vi "Configure Math Function Characteristics.vi"(0 "VISA resource name":refnum<visa-resource-name>, 1 "Vertical Offset (0.0)":dbl, 2 "Vertical Scale (10.0)":dbl=10.0, 3 "Integrate DC Offset (0.0)":dbl, 5 "Math Operation (0: Add)":i32(ring) items=["Add", "Subtract", "Multiply", "Integrate", "Diff", "FFT", "SQRT", "Magnify", "Absolute", "Square", "LN", "LOG", "EXP", "TEN", "Lowpass", "Highpass", "Divide", "Linear", "Trend", "Btiming", "Bstate", "Envelope", "Smoothing", "Max Hold", "Min Hold", "Average", "Clock Recovery", "Peak", "FFT Phase", "MAX", "MIN", "Bandpass", "Serchart"], 7 "GOFT Math Operation (0: Add)":i32(ring) items=["Add", "Subtract", "Multiply"], 9 "Enable Display (T: Enable)":bool=TRUE, 11 "error in (no error)":errorcluster, 12 "Vertical Range (8.0 V)":dbl=8.0, 13 "Vertical Scale Units (0: V)":i32(ring) items=["V", "dB"], 14 "Math Function Index (1: Math Function 1)":i32(ring)=1 items=["Math Function 1"=1, "Math Function 2"=2, "Math Function 3"=3, "Math Function 4"=4]) -> (4 "VISA resource name out":refnum<visa-resource-name>, 15 "error out":errorcluster)   [LabVIEW 2017, in "Agilent 2000 3000 X-Series.lvlib"]
doc: "Configures the math function."
uses:
  Agilent 2000 3000 X-Series.lvlib
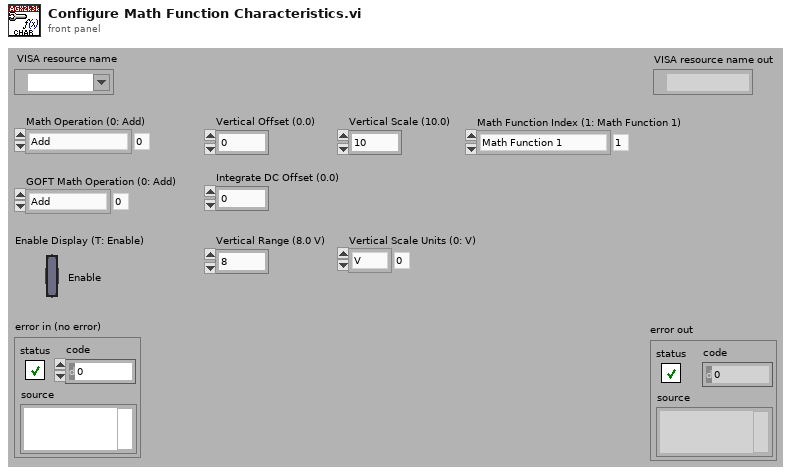
[diagram p1: front panel]
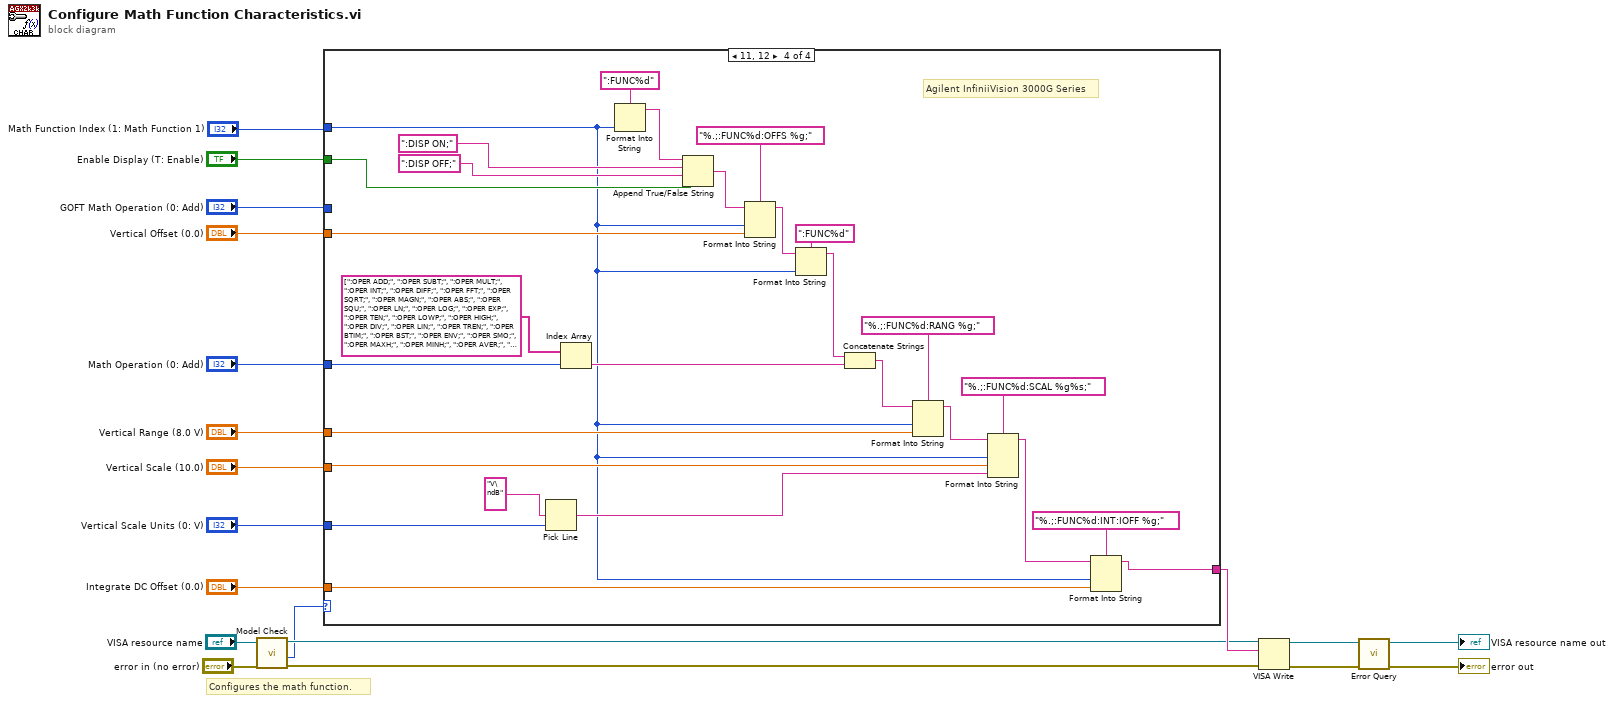
[diagram p0: block diagram]
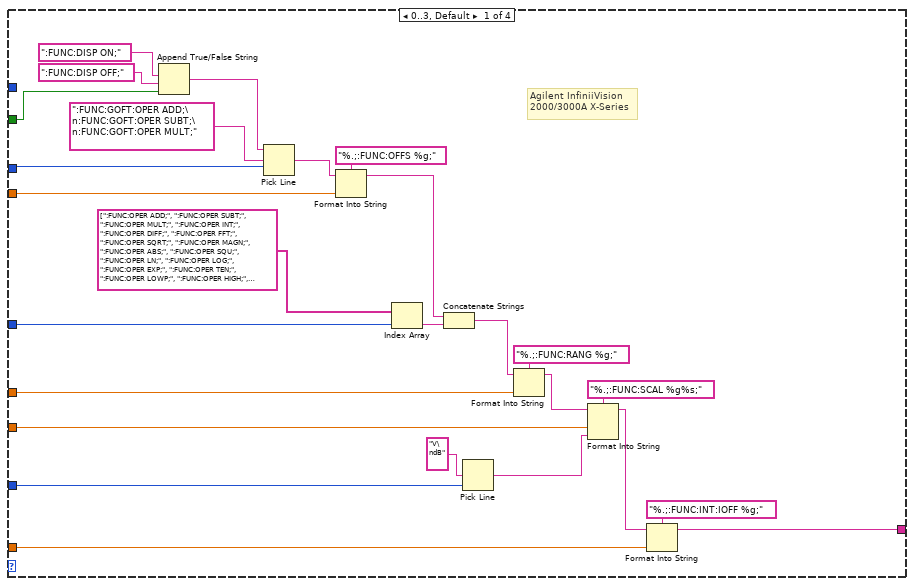
[diagram p2: hidden frame]
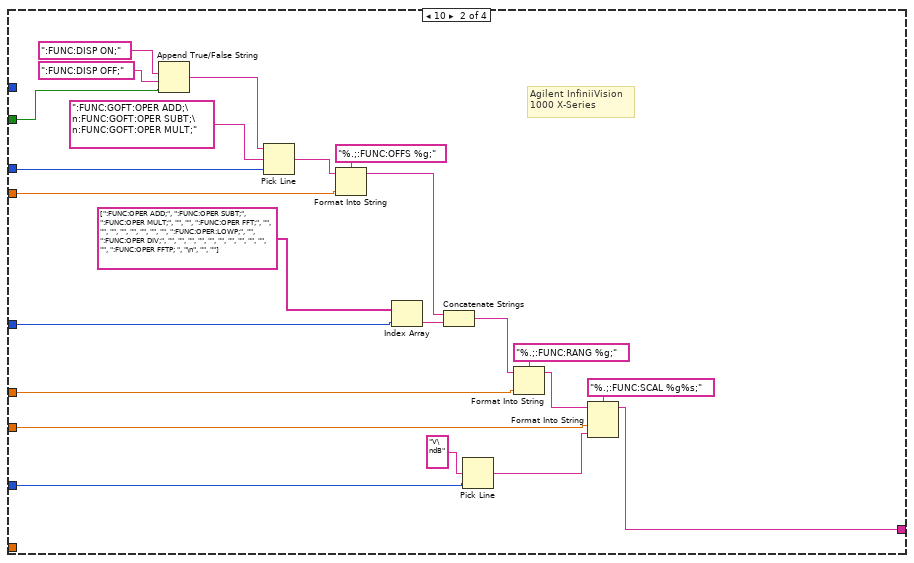
[diagram p3: hidden frame]
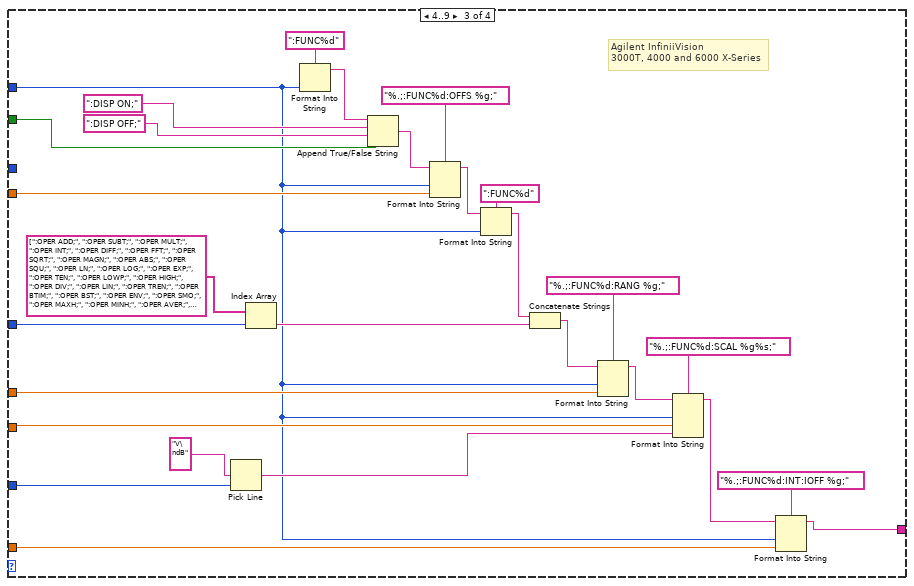
[diagram p4: hidden frame]
diagram:
  # "Configures the math function."
  n1 = call "Model Check.vi"("error in (no error)"="error in (no error)", "VISA resource name"="VISA resource name") -> ("error out"=w2:errorcluster, "Model"=w1:i32, "VISA resource name out"=w3:refnum<visa-resource-name>)  [unwired: 7 out]
  n2 = case shown="11, 12" w1 {
    tunnel: "Enable Display (T: Enable)" -> [w30 w53 w82 w110]
    tunnel: "GOFT Math Operation (0: Add)" -> [w29 w46 _ _]
    tunnel: "Vertical Offset (0.0)" -> [w28 w52 w81 w109]
    tunnel: "Math Operation (0: Add)" -> [w27 w51 w72 w100]
    tunnel: "Vertical Range (8.0 V)" -> [w26 w50 w80 w108]
    tunnel: "Vertical Scale (10.0)" -> [w25 w49 w77 w105]
    tunnel: "Vertical Scale Units (0: V)" -> [w24 w48 w78 w106]
    tunnel: "Integrate DC Offset (0.0)" -> [w23 _ w76 w104]
    tunnel: "Math Function Index (1: Math Function 1)" -> [_ _ w74 w102]
    tunnel: [w22 w47 w71 w99] -> w6
    frame 0..3, Default {
      # "Agilent InfiniiVision\n2000/3000A X-Series"
      n3 = Append True/False String(1:w30, 2:":FUNC:DISP OFF;", 3:":FUNC:DISP ON;") -> (0:w42:string)  [unwired: 1 out]
      n4 = Pick Line(string ("")=w42, multi-line string=":FUNC:GOFT:OPER ADD;\n:FUNC:GOFT:OPER SUBT;\n:FUNC:GOFT:OPER MULT;", line index=w29) -> (output string=w41:string)
      n5 = Format Into String(format string="%.;:FUNC:OFFS %g;", initial string=w41, w28) -> (resulting string=w34:string)  [unwired: 1 in, 1 out]
      n6 = Index Array(array=string[] [":FUNC:OPER ADD;", ":FUNC:OPER SUBT;", ":FUNC:OPER MULT;", ":FUNC:OPER INT;", ":FUNC:OPER DIFF;", ":FUNC:OPER FFT;", ":FUNC:OPER SQRT;", ":FUNC:OPER MAGN;", ":FUNC:OPER ABS;", ":FUNC:OPER SQU;", ":FUNC:OPER LN;", ":FUNC:OPER LOG;", ":FUNC:OPER EXP;", ":FUNC:OPER TEN;", ":FUNC:OPER LOWP;", ":FUNC:OPER HIGH;", ":FUNC:OPER DIV;", ":FUNC:OPER LIN;", ":FUNC:OPER TREN;", ":FUNC:OPER BTIM;", ":FUNC:OPER BST;", "", "", "", "", "", "", "", "\n", "", ""], index=w27) -> (element=w20:string)
      n7 = Concatenate Strings(w34, w20) -> (w33:string)
      n8 = Pick Line(multi-line string="V\ndB", line index=w24) -> (output string=w35:string)  [unwired: 1 out]
      n9 = Format Into String(format string="%.;:FUNC:RANG %g;", initial string=w33, w26) -> (resulting string=w37:string)  [unwired: 1 in, 1 out]
      n10 = Format Into String(format string="%.;:FUNC:SCAL %g%s;", initial string=w37, w25, w35) -> (resulting string=w31:string)  [unwired: 1 in, 1 out]
      n11 = Format Into String(format string="%.;:FUNC:INT:IOFF %g;", initial string=w31, w23) -> (resulting string=w22:string)  [unwired: 1 in, 1 out]
    }
    frame 10 {
      # "Agilent InfiniiVision\n1000 X-Series"
      n12 = Append True/False String(1:w53, 2:":FUNC:DISP OFF;", 3:":FUNC:DISP ON;") -> (0:w65:string)  [unwired: 1 out]
      n13 = Pick Line(string ("")=w65, multi-line string=":FUNC:GOFT:OPER ADD;\n:FUNC:GOFT:OPER SUBT;\n:FUNC:GOFT:OPER MULT;", line index=w46) -> (output string=w64:string)
      n14 = Format Into String(format string="%.;:FUNC:OFFS %g;", initial string=w64, w52) -> (resulting string=w57:string)  [unwired: 1 in, 1 out]
      n15 = Index Array(array=string[] [":FUNC:OPER ADD;", ":FUNC:OPER SUBT;", ":FUNC:OPER MULT;", "", "", ":FUNC:OPER FFT;", "", "", "", "", "", "", "", "", ":FUNC:OPER:LOWP;", "", ":FUNC:OPER DIV;", "", "", "", "", "", "", "", "", "", "", "", ":FUNC:OPER FFTP; ", "\n", "", ""], index=w51) -> (element=w54:string)
      n16 = Concatenate Strings(w57, w54) -> (w56:string)
      n17 = Pick Line(multi-line string="V\ndB", line index=w48) -> (output string=w58:string)  [unwired: 1 out]
      n18 = Format Into String(format string="%.;:FUNC:RANG %g;", initial string=w56, w50) -> (resulting string=w60:string)  [unwired: 1 in, 1 out]
      n19 = Format Into String(format string="%.;:FUNC:SCAL %g%s;", initial string=w60, w49, w58) -> (resulting string=w47:string)  [unwired: 1 in, 1 out]
    }
    frame 4..9 {
      # "Agilent InfiniiVision\n3000T, 4000 and 6000 X-Series"
      n20 = Pick Line(multi-line string="V\ndB", line index=w78) -> (output string=w79:string)  [unwired: 1 out]
      n21 = Index Array(array=string[] [":OPER ADD;", ":OPER SUBT;", ":OPER MULT;", ":OPER INT;", ":OPER DIFF;", ":OPER FFT;", ":OPER SQRT;", ":OPER MAGN;", ":OPER ABS;", ":OPER SQU;", ":OPER LN;", ":OPER LOG;", ":OPER EXP;", ":OPER TEN;", ":OPER LOWP;", ":OPER HIGH;", ":OPER DIV;", ":OPER LIN;", ":OPER TREN;", ":OPER BTIM;", ":OPER BST;", ":OPER ENV;", ":OPER SMO;", ":OPER MAXH;", ":OPER MINH;", ":OPER AVER;", ":OPER CLOCK;", ":OPER PEAK; ", ":OPER FFTP;\n", ":OPER MAX;", ":OPER MIN;"], index=w72) -> (element=w88:string)
      n22 = Format Into String(format string=":FUNC%d", w74) -> (resulting string=w83:string)  [unwired: 2 in, 1 out]
      n23 = Append True/False String(1:w82, 2:":DISP OFF;", 3:":DISP ON;", 4:w83) -> (0:w70:string)
      n24 = Format Into String(format string="%.;:FUNC%d:OFFS %g;", initial string=w70, w74, w81) -> (resulting string=w69:string)  [unwired: 1 in, 1 out]
      n25 = Format Into String(format string=":FUNC%d", initial string=w69, w74) -> (resulting string=w73:string)  [unwired: 1 in, 1 out]
      n26 = Concatenate Strings(w73, w88) -> (w87:string)
      n27 = Format Into String(format string="%.;:FUNC%d:RANG %g;", initial string=w87, w74, w80) -> (resulting string=w91:string)  [unwired: 1 in, 1 out]
      n28 = Format Into String(format string="%.;:FUNC%d:SCAL %g%s;", initial string=w91, w74, w77, w79) -> (resulting string=w85:string)  [unwired: 1 in, 1 out]
      n29 = Format Into String(format string="%.;:FUNC%d:INT:IOFF %g;", initial string=w85, w74, w76) -> (resulting string=w71:string)  [unwired: 1 in, 1 out]
    }
    frame 11, 12 {
      # "Agilent InfiniiVision 3000G Series"
      n30 = Pick Line(multi-line string="V\ndB", line index=w106) -> (output string=w107:string)  [unwired: 1 out]
      n31 = Index Array(array=string[] [":OPER ADD;", ":OPER SUBT;", ":OPER MULT;", ":OPER INT;", ":OPER DIFF;", ":OPER FFT;", ":OPER SQRT;", ":OPER MAGN;", ":OPER ABS;", ":OPER SQU;", ":OPER LN;", ":OPER LOG;", ":OPER EXP;", ":OPER TEN;", ":OPER LOWP;", ":OPER HIGH;", ":OPER DIV;", ":OPER LIN;", ":OPER TREN;", ":OPER BTIM;", ":OPER BST;", ":OPER ENV;", ":OPER SMO;", ":OPER MAXH;", ":OPER MINH;", ":OPER AVER;", "", ":OPER PEAK; ", ":OPER FFTP;\n", ":OPER MAX;", ":OPER MIN;", ":OPER BAND; ", ":OPER SERC; "], index=w100) -> (element=w116:string)
      n32 = Format Into String(format string=":FUNC%d", w102) -> (resulting string=w111:string)  [unwired: 2 in, 1 out]
      n33 = Append True/False String(1:w110, 2:":DISP OFF;", 3:":DISP ON;", 4:w111) -> (0:w98:string)
      n34 = Format Into String(format string="%.;:FUNC%d:OFFS %g;", initial string=w98, w102, w109) -> (resulting string=w97:string)  [unwired: 1 in, 1 out]
      n35 = Format Into String(format string=":FUNC%d", initial string=w97, w102) -> (resulting string=w101:string)  [unwired: 1 in, 1 out]
      n36 = Concatenate Strings(w101, w116) -> (w115:string)
      n37 = Format Into String(format string="%.;:FUNC%d:RANG %g;", initial string=w115, w102, w108) -> (resulting string=w119:string)  [unwired: 1 in, 1 out]
      n38 = Format Into String(format string="%.;:FUNC%d:SCAL %g%s;", initial string=w119, w102, w105, w107) -> (resulting string=w113:string)  [unwired: 1 in, 1 out]
      n39 = Format Into String(format string="%.;:FUNC%d:INT:IOFF %g;", initial string=w113, w102, w104) -> (resulting string=w99:string)  [unwired: 1 in, 1 out]
    }
  }
  n40 = VISA Write(VISA resource name=w3, write buffer=w6, error in (no error)=w2) -> (VISA resource name out=w19:refnum<visa-resource-name>, error out=w18:errorcluster)  [unwired: 1 out]
  n41 = call "Error Query.vi"("error in (no error)"=w18, "VISA resource name"=w19) -> ("error out"=→"error out":errorcluster, "VISA resource name out"=→"VISA resource name out":refnum<visa-resource-name>)  [unwired: 8 out]
